vi "Bohman Window (DBL).vi"(11 "X":dbl[](array[numeric])) -> (0 "error":i32, 3 "Windowed X":dbl[](array[numeric]))   [LabVIEW 2024, in "NI_AALPro.lvlib"]
doc: "<p>Applies a Bohman window to the input signal <strong>X</strong>. Wire data to the <strong>X</strong> input to determine the polymorphic instance to use or <a href=\"nihelplauncher://docs/csh?context=lvcore_lvhowto_selectingdefaultinstpolyvi\">manually select</a> the instance.</p>"
uses:
  NI_AALPro.lvlib
  <resource>/lvanlys.dll
panel:
  # "Bohman Window"
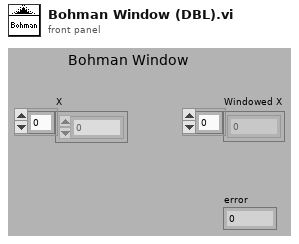
[diagram p1: front panel]
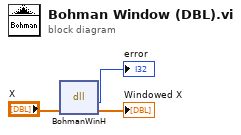
[diagram p0: block diagram]
diagram:
  n1 = dll-call lib="C:/Program Files (x86)/National Instruments/LabVIEW 2024/resource/lvanlys.*" fn="BohmanWinH"("X"="X") -> ("error"=→"error":i32, "X"=→"Windowed X":dbl[])  [unwired: 3 in, 2 out]
